vi "Module Type.vi"(11 "Redlines Module in":refnum<class "Redlines Module.lvclass">) -> (2 "Module Type":string)   [LabVIEW 2020, in "VolatusData.lvlib" / "Redlines Module.lvclass"]
uses:
  Redlines Module.lvclass
  Redlines Module.lvclass/Redlines Module.ctl
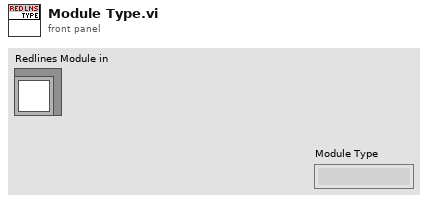
[diagram p1: front panel]
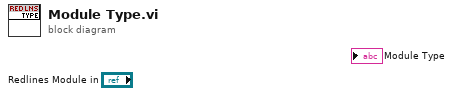
[diagram p0: block diagram]
diagram:
